vi "Wrt_Ch_States.vi"(7 "ReadOnlyIn":T1={"Qref"={"ValveCTR"=refnum, "Error"=refnum}, "UI_EN"=FALSE, "UserEventREF"={"TimeBasedProducer"={"Reg"=refnum, "Ref"=refnum}, "TimeBasedTempRead"={"Reg"=refnum, "Ref"=refnum}}, "UI_REF"=variant, "Paths"={"Log_Dir"=path "", "TempLog"=path "", "WateringLog"=path "", "Error"=path "", "Settings_Dir"=path "", "CFG.ini"=path "", "Plant_Digital_OP"=path "", "TimeTable"=path "", "Consol_Dir"=path "", "Input"=path "", "Output"=path "", "Timeout"=path "", "TimeoutTable"=path "", "Ch_Stat"=path "", "Temp"=path ""}, "PI_REF"={"IO"=enum."Remote", "Interface"=enum."Serial", "LINX Device Config"={"Interface"=enum."Serial", "COM Port"="", "TCP Configuration"={"IP Address"="", "Port"=0}, "Device Family"=0, "Device ID"=0, "Device Name"="", "TCP Ref"=refnum, "Channels"={"DI"=[], "DO"=[], "AI"=[], "AO"=[], "PWM"=[], "QE"=[], "UART"=[], "I2C 2"=[], "SPI"=[], "CAN"=[], "Servo"=[], "AI Ref (V)"=0.0, "AI Resolution (Bits)"=0, "AO Ref (V)"=0.0, "AO Resolution (Bits)"=0}}}, "CFG"={"ProducerEn_PC"=FALSE, "Producer_PC_ms"=0, "ProducerEn_PI"=FALSE, "Producer_PI_ms"=0, "TempLogInterval"=15, "SystemResetTime"=0.0}} {"CFG"."SystemResetTime" format="%<%H:%M:%S>t"}, 8 "error in (no error)":errorcluster, 11 "Read_Write_Valv_IN":T9 {"ValidCh" items=["7"=7, "11"=11, "12"=12, "13"=13, "15"=15, "16"=16, "18"=18, "29"=29, "32"=32, "33"=33, "35"=35, "36"=36, "37"=37, "38"=38, "40"=40]}) -> (0 "error out":errorcluster, 3 "Read_Write_Valv_OUT":T9 {"ValidCh" items=["7"=7, "11"=11, "12"=12, "13"=13, "15"=15, "16"=16, "18"=18, "29"=29, "32"=32, "33"=33, "35"=35, "36"=36, "37"=37, "38"=38, "40"=40]})   [LabVIEW 2014, in "ValveCTRL.lvlib"]
uses:
  ValveCTRL.lvlib
  TypeDef/Read_Write.ctl
  TypeDef/ChannelStatus.ctl
  TypeDef/CHs_List.ctl
  Main/TypeDef/ReadOnly.ctl
  TypeDef/Queue_Cluster.ctl
  TypeDef/States_Enum.ctl
  Main/TypeDef/EventData.ctl
  <vilib>/MakerHub/LINX/Private/Type Defs/LINX Ref.ctl
  <vilib>/MakerHub/LINX/Private/Type Defs/Platform.ctl
  <vilib>/MakerHub/LINX/Private/Type Defs/Interface.ctl
  <vilib>/MakerHub/LINX/Private/Device/Type Defs/LINX Device Config.ctl
  <vilib>/MakerHub/LINX/Private/Device/Type Defs/TCP Config.ctl
  <vilib>/MakerHub/LINX/Private/Device/Type Defs/Channels.ctl
  Main/Init/ReadInitCFG/TypeDef/CFG_Cluster.ctl
  Main/Main.lvlib
  <vilib>/MakerHub/LINX/LMH-LINX.lvlib
  <vilib>/MakerHub/LINX/Private/Device/Device.lvlib
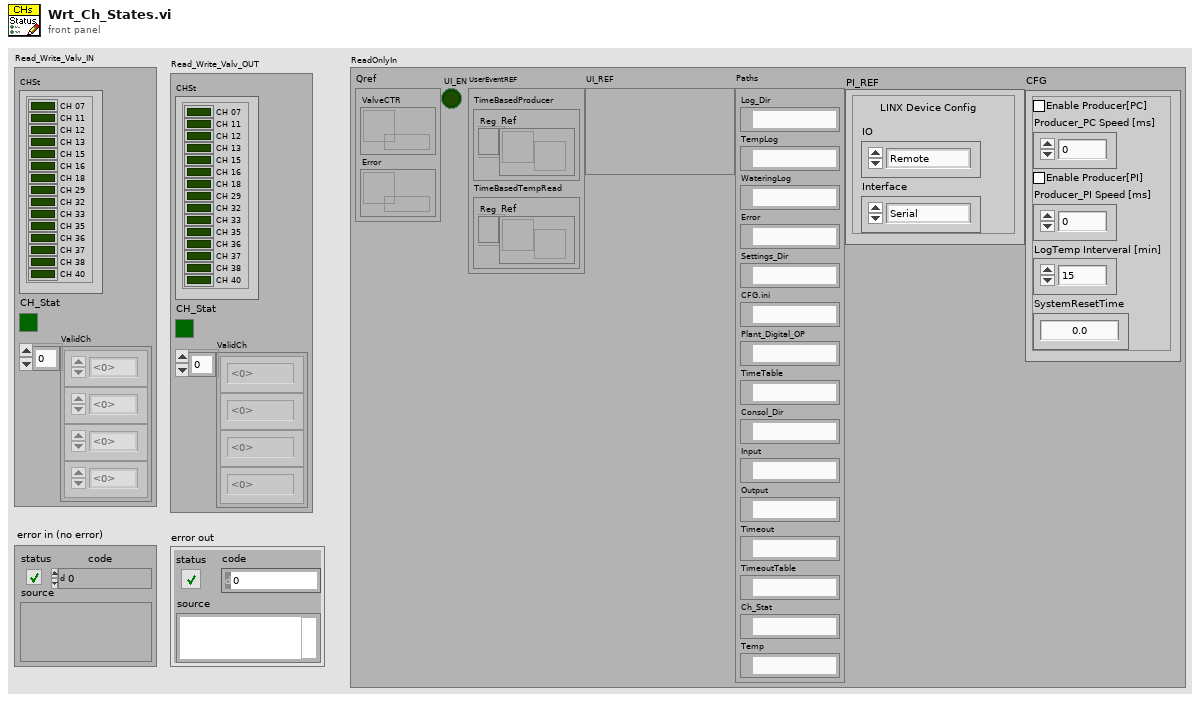
[diagram p1: front panel]
types:
  T1 = typedef "Main.lvlib/ReadOnly.ctl" = cluster{"Qref":cluster{"ValveCTR":refnum<queue>, "Error":refnum<queue>}, "UI_EN":bool, "UserEventREF":cluster{"TimeBasedProducer":cluster{"Reg":refnum<event-registration>, "Ref":refnum<user-event>}, "TimeBasedTempRead":cluster{"Reg":refnum<event-registration>, "Ref":refnum<user-event>}}, "UI_REF":variant, "Paths":cluster{"Log_Dir":path, "TempLog":path, "WateringLog":path, "Error":path, "Settings_Dir":path, "CFG.ini":path, "Plant_Digital_OP":path, "TimeTable":path, "Consol_Dir":path, "Input":path, "Output":path, "Timeout":path, "TimeoutTable":path, "Ch_Stat":path, "Temp":path}, "PI_REF":T2, "CFG":T8}
  T2 = typedef "LMH-LINX.lvlib/LINX Ref.ctl" = cluster{"IO":T3, "Interface":T4, "LINX Device Config":T5}
  T3 = typedef "LMH-LINX.lvlib/Platform.ctl" = enum16{"Remote", "Local"}
  T4 = typedef "LMH-LINX.lvlib/Interface.ctl" = enum16{"Serial", "TCP"}
  T5 = typedef "LMH-LINX.lvlib/Device.lvlib/LINX Device Config.ctl" = cluster{"Interface":T4, "COM Port":refnum<visa-resource-name>, "TCP Configuration":T6, "Device Family":u8, "Device ID":u8, "Device Name":string, "TCP Ref":refnum<k5>, "Channels":T7}
  T6 = typedef "LMH-LINX.lvlib/Device.lvlib/TCP Config.ctl" = cluster{"IP Address":string, "Port":u16}
  T7 = typedef "LMH-LINX.lvlib/Channels.ctl" = cluster{"DI":u8[], "DO":u8[], "AI":u8[], "AO":u8[], "PWM":u8[], "QE":u8[], "UART":u8[], "I2C 2":u8[], "SPI":u8[], "CAN":u8[], "Servo":u8[], "AI Ref (V)":dbl, "AI Resolution (Bits)":u8, "AO Ref (V)":dbl, "AO Resolution (Bits)":u8}
  T8 = typedef "Main.lvlib/CFG_Cluster.ctl" = cluster{"ProducerEn_PC":bool, "Producer_PC_ms":u32, "ProducerEn_PI":bool, "Producer_PI_ms":u32, "TempLogInterval":u32, "SystemResetTime":dbl}
  T9 = typedef "ValveCTRL.lvlib/Read_Write.ctl" = cluster{"CHSt":T10, "CH_Stat":bool, "ValidCh":T11[]}
  T10 = typedef "ValveCTRL.lvlib/ChannelStatus.ctl" = cluster{"CH 07":bool, "CH 11":bool, "CH 12":bool, "CH 13":bool, "CH 15":bool, "CH 16":bool, "CH 18":bool, "CH 29":bool, "CH 32":bool, "CH 33":bool, "CH 35":bool, "CH 36":bool, "CH 37":bool, "CH 38":bool, "CH 40":bool}
  T11 = typedef "ValveCTRL.lvlib/CHs_List.ctl" = u8
  T12 = enum16{"open", "replace", "create", "open or create", "replace or create", "replace or create with confirmation"}
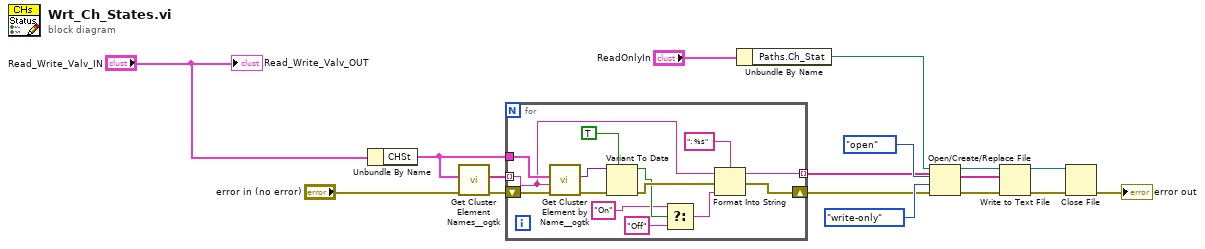
[diagram p0: block diagram]
diagram:
  n1 = Unbundle By Name("Read_Write_Valv_IN") -> ("CHSt"=w3:T10)
  n2 = call <userlib>:"Get Cluster Element Names__ogtk.vi"("error in (no error)"="error in (no error)", "Cluster"=w3) -> ("error out"=w6:errorcluster, "Element Names"=w7:string[])  [unwired: 8 in]
  n3 = for {
    tunnel: w7 -> [w25] mode=indexing
    tunnel: w3 -> [w29]
    tunnel: [w17] -> w8 mode=indexing
    shift-right: [w18] -> w9
    shift-left: w6 -> [w30]
    n4 = call <userlib>:"Get Cluster Element by Name__ogtk.vi"("error in (no error)"=w30, "Element Name"=w25, "Cluster"=w29) -> ("error out"=w28:errorcluster, "VElement"=w27:variant)  [unwired: 6 in, 1 out]
    n5 = Variant To Data(error in=w28, type=TRUE, Variant=w27) -> (data=w23:bool, error out=w24:errorcluster)
    n6 = Select(t="On" ("Data Name"), s=w23, f="Off") -> (s? t:f=w22:string)
    n7 = Format Into String(format string=": %s", initial string=w25, error in=w24, w22) -> (resulting string=w17:string, error out=w18:errorcluster)
  }
  n8 = Unbundle By Name("ReadOnlyIn") -> ("Paths.Ch_Stat"=w1:path)
  n9 = Open/Create/Replace File(file path (use dialog)=w1, error in=w9, operation (0:open)=T12."open", access (0:read/write)=enum16{"read/write", "read-only", "write-only"}."write-only") -> (refnum out=w11:refnum<file>, error out=w10:errorcluster)  [unwired: 2 in, 1 out]
  n10 = Write to Text File(file (use dialog)=w11, text=w8, error in=w10) -> (refnum out=w15:refnum<file>, error out=w14:errorcluster)  [unwired: 1 in, 1 out]
  n11 = Close File(refnum=w15, error in=w14) -> (error out=→"error out":errorcluster)  [unwired: 1 out]
  "Read_Write_Valv_OUT" <- "Read_Write_Valv_IN"
